vi "2AntennaAcq.vi"(0 "IVI Refnum in":refnum<k15>, 5 "samples per acquisition":i32, 9 "Carrier":dbl, 11 "error in (no error)":errorcluster) -> (4 "IVI Refnum out":refnum<k15>, 6 "data":cdb[][](array[numeric]), 15 "error out":errorcluster)   [LabVIEW 2015]
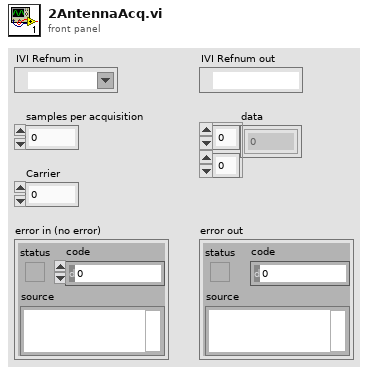
[diagram p1: front panel]
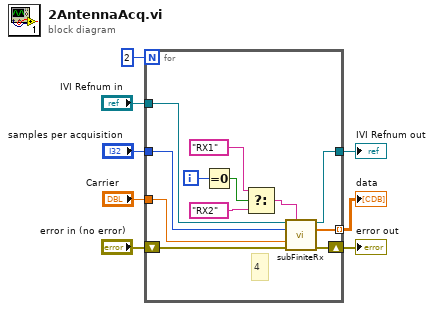
[diagram p0: block diagram]
diagram:
  n1 = for {
    N: 2 -> [_]
    tunnel: "IVI Refnum in" -> [w20]
    tunnel: [w19] -> w2
    tunnel: "Carrier" -> [w17]
    tunnel: "samples per acquisition" -> [w16]
    tunnel: [w14] -> w8 mode=indexing
    shift-right: [w15] -> w6
    shift-left: "error in (no error)" -> [w18]
    i -> [w13]
    # "4"
    n2 = Equal To 0?(x=w13) -> (x = 0?=w12:bool)
    n3 = Select(t="RX1" ("Active Antenna"), s=w12, f="RX2" ("Active Antenna")) -> (s? t:f=w9:string)
    n4 = call "subFiniteRx.vi"("IVI Refnum in"=w20, "Active Antenna"=w9, "Number of Samples"=w16, "Carrier Frequency"=w17, "error in (no error)"=w18) -> ("IVI Refnum out"=w19:refnum<k15>, "data"=w14:cdb[], "error out"=w15:errorcluster)  [unwired: 8 in]
  }
  "data" <- w8
  "error out" <- w6
  "IVI Refnum out" <- w2
